vi "MainPanel.vi"() -> ()   [LabVIEW 2023]
panel:
  in  "vi path":path
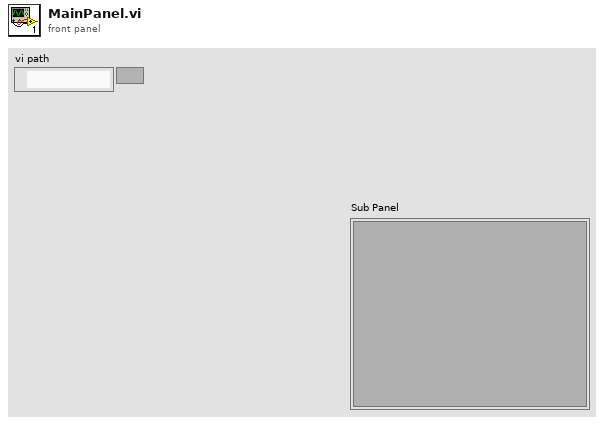
[diagram p1: front panel]
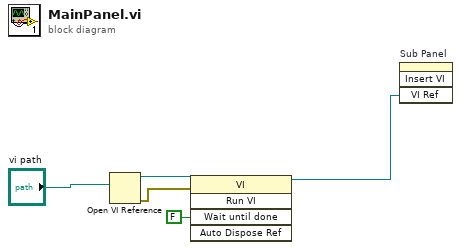
[diagram p0: block diagram]
diagram:
  n1 = Open VI Reference(vi path="vi path") -> (vi reference=w4:refnum<vi>, error out=w3:errorcluster)  [unwired: 5 in]
  n2 = invoke class="VI" method="Run VI"(reference=w4, error in=w3, "Wait until done"=FALSE ("Wait Until Done")) -> (reference out=w2:refnum<vi>)  [unwired: 2 in, 4 out]
  n3 = invoke on="Sub Panel" class="SubPnl" method="Insert VI"("VI Ref"=w2) -> ()  [unwired: 3 in, 4 out]
